vi "Keyboard Test.vi"(3 "Input buffer":T3, 4 "Sequence Context":T1) -> (0 "error out":errorcluster, 1 "Test Data":T2 {"Numeric Measurement" format="%.2f"})   [LabVIEW 2011]
uses:
  SupportVIs.llb/LabVIEW Test - Input Buffer.ctl
  <vilib>/addons/TestStand/_TSLegacy.llb/LabVIEW Test - Test Data.ctl
  <vilib>/addons/TestStand/_TSLegacy.llb/LabVIEW Test - Sequence Context.ctl
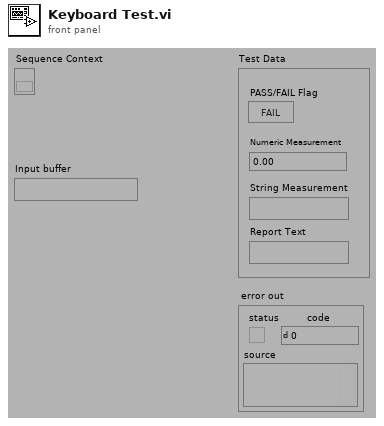
[diagram p1: front panel]
types:
  T1 = typedef "LabVIEW Test - Sequence Context.ctl" = refnum<k7>
  T2 = typedef "LabVIEW Test - Test Data.ctl" = cluster{"PASS/FAIL Flag":bool, "Numeric Measurement":dbl, "String Measurement":string, "Report Text":string}
  T3 = typedef "LabVIEW Test - Input Buffer.ctl" = string
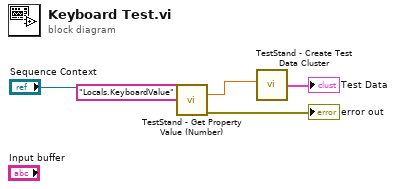
[diagram p0: block diagram]
diagram:
  n1 = call "TestStand - Get Property Value (Number).vi"("Sequence Context In"="Sequence Context", "Lookup String"="Locals.KeyboardValue" ("lookupString")) -> ("Value"=w2:dbl, "error out"=→"error out":errorcluster)  [unwired: 1 in, 11 out]
  n2 = call "TestStand - Create Test Data Cluster.vi"("Numeric Measurement"=w2) -> ("Test Data"=→"Test Data":T2)  [unwired: 3 in]
